vi "Simulation Initialize.vi"(0 "simulation configuration":T1={"maxTime"=5.0, "enableVisualization"=TRUE, "Environment Definition"=path "iRobot Navigation State Machine.vi", "Record Location"=path "Simulation Record.xml", "autograde?"=TRUE, "interactive?"=FALSE, "Feedback Mode"=enum."debug navigation", "Robot State Charts"=[path "C:/Users/blueuser/Desktop/Robo Sim Berkley/cpsgrader-release-0.4/Simulators/EECS149lab/src/LabVIEW/statechart/Simulation Statechart.vi"], "statechart"=path "C:/Users/blueuser/Desktop/Robo Sim Berkley/cpsgrader-release-0.4/Simulators/EECS149lab/src/LabVIEW/statechart/Simulation Statechart.vi"}, 2 "Statechart display":refnum<vi>, 3 "Simulator display":refnum<vi>, 5 "Real Time":bool, 11 "Error In":errorcluster) -> (4 "simulator":T3={"configuration"={"maxTime"=5.0, "enableVisualization"=TRUE, "Environment Definition"=path "iRobot Navigation State Machine.vi", "Record Location"=path "Simulation Record.xml", "autograde?"=TRUE, "interactive?"=FALSE, "Feedback Mode"=enum."debug navigation", "Robot State Charts"=[path "C:/Users/blueuser/Desktop/Robo Sim Berkley/cpsgrader-release-0.4/Simulators/EECS149lab/src/LabVIEW/statechart/Simulation Statechart.vi"], "statechart"=path "C:/Users/blueuser/Desktop/Robo Sim Berkley/cpsgrader-release-0.4/Simulators/EECS149lab/src/LabVIEW/statechart/Simulation Statechart.vi"}, "Statechart\ndisplay"=refnum, "first step?"=FALSE, "Robots Simulation Statecharts"=[], "Robots"=[]}, 15 "Error Out":errorcluster)   [LabVIEW 2015]
uses:
  Simulator.ctl
  CyberSim interface/Simulation Configuration.ctl
  autograder/feedbackMode.ctl
  Multi Bot Code/RobotData.ctl
  <instrlib>/DC Motor Controller/HAIOL/DC Motor Controller.lvclass
  Simulation Trace Operation.ctl
  Simulation Call Statechart Operation.ctl
  <vilib>/robotics/Simulator/Engine/ctl/Simulation Mode.ctl
  <vilib>/robotics/Simulator/Engine/ctl/Step Mode.ctl
  <vilib>/robotics/Simulator/NI_Robotics_Simulator.lvlib
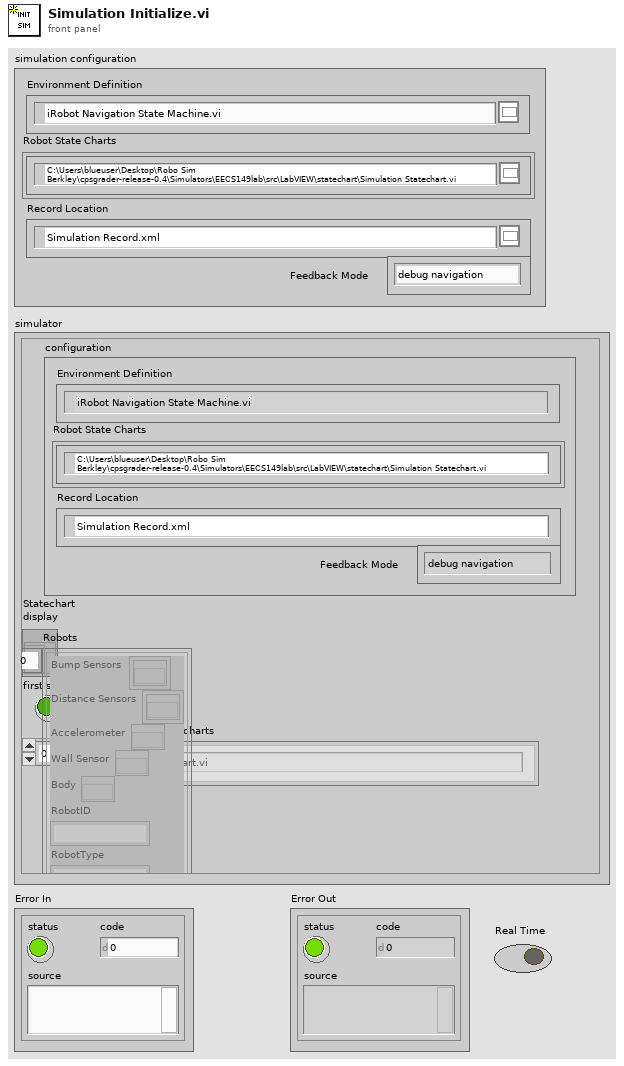
[diagram p1: front panel]
types:
  T1 = typedef "Simulation Configuration.ctl" = cluster{"maxTime":sgl, "enableVisualization":bool, "Environment Definition":path, "Record Location":path, "autograde?":bool, "interactive?":bool, "Feedback Mode":T2, "Robot State Charts":path[], "statechart":path}
  T2 = typedef "feedbackMode.ctl" = enum32{"debug navigation", "debug hill climb", "autograde navigation", "autograde hill climb"}
  T3 = typedef "Simulator.ctl" = cluster{"configuration":T1, "Statechart\ndisplay":refnum<vi>, "first step?":bool, "Robots Simulation Statecharts":path[], "Robots":T4[]}
  T4 = typedef "RobotData.ctl" = cluster{"Bump Sensors":refnum<k20>[], "Distance Sensors":refnum<k20>[], "Accelerometer":refnum<k20>, "Wall Sensor":refnum<k20>, "Body":refnum<k20>, "RobotID":string, "RobotType":string, "Left Motor":refnum<class "DC Motor Controller.lvclass">, "Right Motor":refnum<class "DC Motor Controller.lvclass">}
  T5 = typedef "NI_Robotics_Simulator.lvlib/Step Mode.ctl" = u16
  T6 = typedef "NI_Robotics_Simulator.lvlib/Simulation Mode.ctl" = u16
  T7 = typedef "Simulation Call Statechart Operation.ctl" = enum16{"Initialize", "Call Statechart", "Finalize"}
  T8 = typedef "Simulation Trace Operation.ctl" = enum16{"Initialize", "Record Trace Element", "Get Trace"}
  T9 = typedef "SimulationIDs.ctl" = cluster{"RobotID":string, "SensorsIDs":string[], "MotorIDs":string[], "RobotType":string}
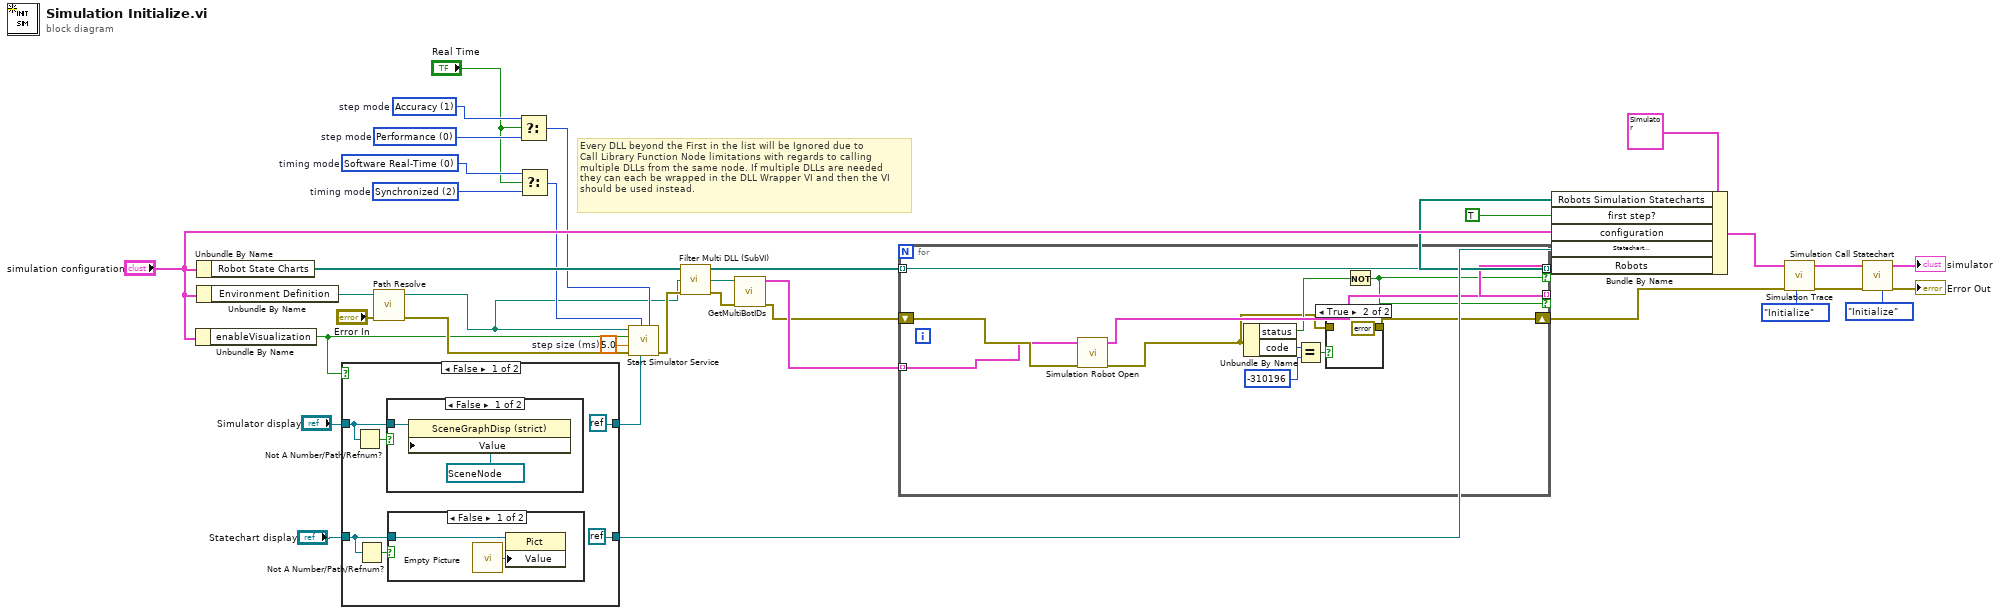
[diagram p0: block diagram]
diagram:
  w9 = T5 1 items=["Performance", "Accuracy"]  # step mode
  w8 = T6 0 items=["Software Real-Time", "Free Running", "Synchronized"]  # timing mode
  w11 = T5 0 items=["Performance", "Accuracy"]  # step mode
  w10 = T6 2 items=["Software Real-Time", "Free Running", "Synchronized"]  # timing mode
  w31 = 5.0  # step size (ms)
  # "Every DLL beyond the First in the list will be Ignored due to \nCall Library Function Node limitations with regards to calling\nmultiple DLLs from the same node. If multiple DLLs are needed\nthey can each be wrapped in the DLL Wrapper VI and then the VI\nshould be used instead."
  n1 = Unbundle By Name("simulation configuration") -> ("enableVisualization"=w27:bool)
  n2 = Unbundle By Name("simulation configuration") -> ("Robot State Charts"=w14:path[])
  n3 = Unbundle By Name("simulation configuration") -> ("Environment Definition"=w34:path)
  n4 = case shown="False" w27 {
    tunnel: "Simulator display" -> [w40 w48]
    tunnel: [refnum<k0> refnum w48] -> w25
    tunnel: "Statechart display" -> [w38 w47]
    tunnel: [refnum<k0> refnum w47] -> w23
    frame False {
      n5 = Not A Number/Path/Refnum?(number/path/refnum=w40) -> (NaN/Path/Refnum?=w41:bool)
      n6 = Not A Number/Path/Refnum?(number/path/refnum=w38) -> (NaN/Path/Refnum?=w39:bool)
      n7 = case shown="False" w41 {
        tunnel: w40 -> [w46 _]
        frame False {
          n8 = property class="SceneGraphDisp (strict)"(reference=w46, "Value"=refnum<vi> refnum ("3D Picture")) -> ()  [unwired: 1 in, 2 out]
        }
        frame True {
        }
      }
      n9 = case shown="False" w39 {
        tunnel: w38 -> [w44 _]
        frame False {
          n10 = call "Empty Picture"() -> ("empty picture"=w43:picture)
          n11 = property class="Pict"(reference=w44, "Value"=w43) -> ()  [unwired: 1 in, 2 out]
        }
        frame True {
        }
      }
    }
    frame True {
    }
  }
  n12 = call "Path Resolve.vi"("Error In"="Error In", "absolute or relative path"=w34) -> ("Error Out"=w33:errorcluster, "resolved path"=w4:path)  [unwired: 8 in]
  n13 = Select(t=w9, s="Real Time", f=w11) -> (s? t:f=w7:T5)
  n14 = Select(t=w8, s="Real Time", f=w10) -> (s? t:f=w6:T6)
  n15 = call <vilib>:"Start Simulator Service.vi"("step mode"=w7, "3D picture refnum"=w25, "timing mode"=w6, "error in (no error)"=w33, "step size (ms)"=w31, "enable 3D visualization (T)"=w27, "manifest file"=w4) -> ("error out"=w12:errorcluster)  [unwired: 4 in]
  n16 = call "Filter Multi DLL (SubVI).vi"("error in (no error)"=w12, "Robot State Charts In"=w14) -> ("error out"=w2:errorcluster, "Robot State Charts Out"=w13:path[])  [unwired: 8 in]
  n17 = call "GetMultiBotIDs.vi"("error in (no error)"=w2, "manifest file"=w4) -> ("error out"=w1:errorcluster, "Array"=w3:T9[])  [unwired: 8 in]
  n18 = for {
    tunnel: w13 -> [w57] mode=indexing
    tunnel: [w59] -> w15 mode=indexing if=w55
    tunnel: [w57] -> w17 mode=indexing if=w55
    shift-right: [w50] -> w16
    shift-left: w1 -> [w58]
    tunnel: w3 -> [w49] mode=indexing
    n19 = call "Simulation Robot Open.vi"("error in (no error)"=w58, "RoboSimIDs"=w49) -> ("error out"=w51:errorcluster, "Robot"=w59:T4)  [unwired: 7 in, 1 out]
    n20 = Unbundle By Name(w51) -> ("status"=w56:bool, "code"=w53:i32)
    n21 = Equal?(x=w53, y=-310196) -> (x = y?=w52:bool)
    n22 = case shown="True" w52 {
      tunnel: w51 -> [w60 _]
      tunnel: [w60 errorcluster {"status"=FALSE, "code"=0, "source"=""} ("error out")] -> w50
      frame False {
      }
      frame True {
      }
    }
    n23 = Not(x=w56) -> (.not. x?=w55:bool)
  }
  n24 = Bundle By Name(cluster=T3 {"configuration"={"maxTime"=5.0, "enableVisualization"=TRUE, "Environment Definition"=path "iRobot Navigation State Machine.vi", "Record Location"=path "Simulation Record.xml", "autograde?"=TRUE, "interactive?"=FALSE, "Feedback Mode"=enum."debug navigation", "Robot State Charts"=[path "C:/Users/blueuser/Desktop/Robo Sim Berkley/cpsgrader-release-0.4/Simulators/EECS149lab/src/LabVIEW/statechart/Simulation Statechart.vi"], "statechart"=path "C:/Users/blueuser/Desktop/Robo Sim Berkley/cpsgrader-release-0.4/Simulators/EECS149lab/src/LabVIEW/statechart/Simulation Statechart.vi"}, "Statechart\ndisplay"=refnum, "first step?"=FALSE, "Robots Simulation Statecharts"=[], "Robots"=[]} ("simulator 2"), "Robots Simulation Statecharts"=w17, "first step?"=TRUE, "configuration"="simulation configuration", "Statechart\ndisplay"=w23, "Robots"=w15) -> (w32:T3)
  n25 = call "Simulation Trace.vi"("operation"=Simulation_Trace_Operation."Initialize", "error in"=w16, "simulator"=w32) -> ("error out"=w29:errorcluster, "simulator"=w30:T3)  [unwired: 5 in, 2 out]
  n26 = call "Simulation Call Statechart.vi"("operation"=Simulation_Call_Statechart_Operation."Initialize", "error in"=w29, "simulator"=w30) -> ("error out"=→"Error Out":errorcluster, "simulator"=→"simulator":T3)  [unwired: 6 in, 1 out]
